vi "FPGA Main.vi"() -> ()   [LabVIEW 2024]
uses:
  <vilib>/eio/EIONode/EIONode.xnode
  <vilib>/rvi/eio/common/nirviEmuTemplateMethod_errors.vi
  Type Definitions/FPGA IO.ctl
  <vilib>/rvi/DataTransferAndStorage/Container/XNode/niFpgaContainer.xnode
  <vilib>/rvi/FIFO/Fifo_Resource/nirvififoEmulationRead.vi
  <vilib>/Platform/TimedLoop/XDataNode/wakeup.ctl
  <vilib>/Platform/TimedLoop/XDataNode/XDNodeRunTimeDep.lvlib
  <vilib>/Platform/TimedLoop/XDataNode/nitl_modes.ctl
  <vilib>/Platform/TimedLoop/XDataNode/timing_clust.ctl
  <vilib>/Platform/TimedLoop/XDataNode/XDataNode.xnode
  <vilib>/rvi/FIFO/Fifo_Resource/nirvififoEmulationWrite.vi
panel:
  in  "Enable Sinewave":bool
  in  "Sinewave Settings":T1={"Frequency (periods/tick)"=0.0, "Phase offset (periods)"=0.0, "Scale factor"=0.999969482421875, "Amplitude offset"=0.0}
  in  "Desired loop rate (ticks)":u32=2666666 caption="Update Interval (Ticks)"
  out "Actual loop rate":u32
  out "Sampling rate achieved?":bool
  out "Measured Period (Ticks)":u32
  out "Low Period (Ticks)":u32
  out "High Period (Ticks)":u32
  in  "Enable PWM":bool
  in  "Squarewave Settings":T2={"Frequency (periods/tick)"=0.0, "Phase offset (periods)"=0.0, "duty cycle (periods)"=0.5}
  in  "Initialize":bool
  in  "Voltage Out":fxp<+/-,20,5> format="%#.3g"
  in  "DO2":bool
  in  "DO1":bool
  in  "STOP FPGA":bool
  out "Potentiometer":fxp<+,18,3> format="%#.14g"
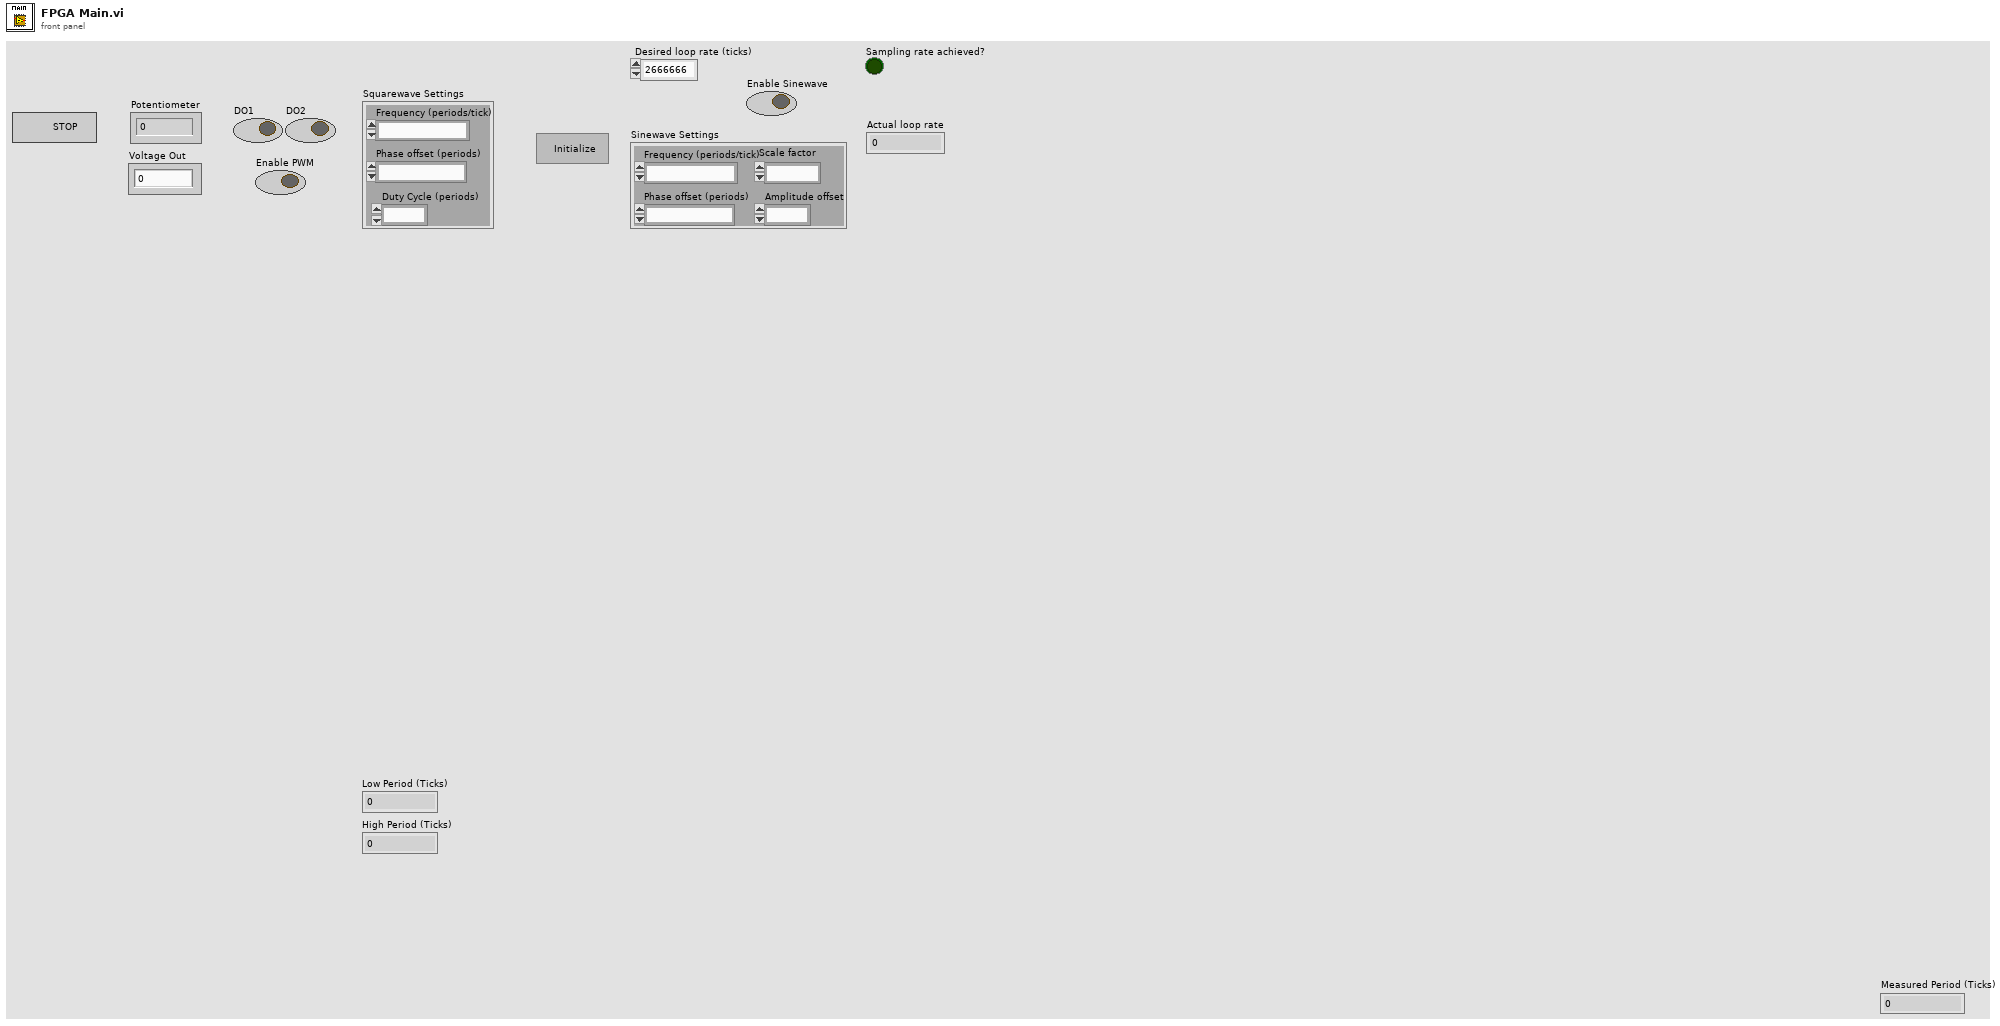
[diagram p1: front panel]
types:
  T1 = cluster{"Frequency (periods/tick)":fxp<+,32,0>, "Phase offset (periods)":fxp<+,32,0>, "Scale factor":fxp<+/-,16,1>, "Amplitude offset":fxp<+/-,16,16>}
  T2 = cluster{"Frequency (periods/tick)":fxp<+,32,0>, "Phase offset (periods)":fxp<+,32,0>, "duty cycle (periods)":fxp<+,32,0>}
  T3 = typedef "FPGA IO.ctl" = cluster{"DO1":bool, "DO2":bool, "Voltage Out":fxp<+/-,20,5>, "Crank Angle":fxp<+,18,3>, "Enable PWM":bool, "Enable Sinewave":bool}
  T4 = cluster{"DO1":bool, "DO2":bool, "Voltage Out":bool, "Crank Angle":bool, "Enable PWM":bool, "Enable Sinewave":bool}
  T5 = typedef "XDNodeRunTimeDep.lvlib/timing_clust.ctl" = cluster{"Expected End [f-1]":u64, "Actual End [f-1]":u64, "Finished Late? [f-1]":bool, "Expected End [i-1]":u64, "Actual End [i-1]":u64, "Finished Late? [i-1]":bool, "Expected Start [i]":u64, "Actual Start [i]":u64, "Expected Start [f]":u64, "Actual Start [f]":u64, "Source Name":string, "Structure Name":string, "Period":i64, "Deadline":i64, "Offset":i64, "Start":i64, "Priority":i32, "Timeout":i32, "Mode":T6, "Wakeup Reason":T7, "Error":errorcluster, "Source Type":string, "Secondary Source Type":string, "Global End Time":u64, "Global Start Time":u64, "Frame Duration":u64, "Iteration Duration":u64, "Assigned CPU":i32, "I/O Scan Engine Mode":u32}
  T6 = typedef "XDNodeRunTimeDep.lvlib/nitl_modes.ctl" = enum32{"No Change", "Process missed periods, maintain original phase", "Discard missed periods, maintain original phase", "Process missed periods, ignore original phase", "Discard missed periods, ignore original phase"}
  T7 = typedef "XDNodeRunTimeDep.lvlib/wakeup.ctl" = enum32{"Normal", "Aborted", "Asynchronous wakeup", "Timing source error", "Timed loop error", "Timeout"}
  T8 = cluster{"DO1":bool, "DO2":bool, "Voltage Out":fxp<+/-,20,5>, "Crank Angle":fxp<+,18,3>, "Enable PWM":bool, "Enable Sinewave":bool}
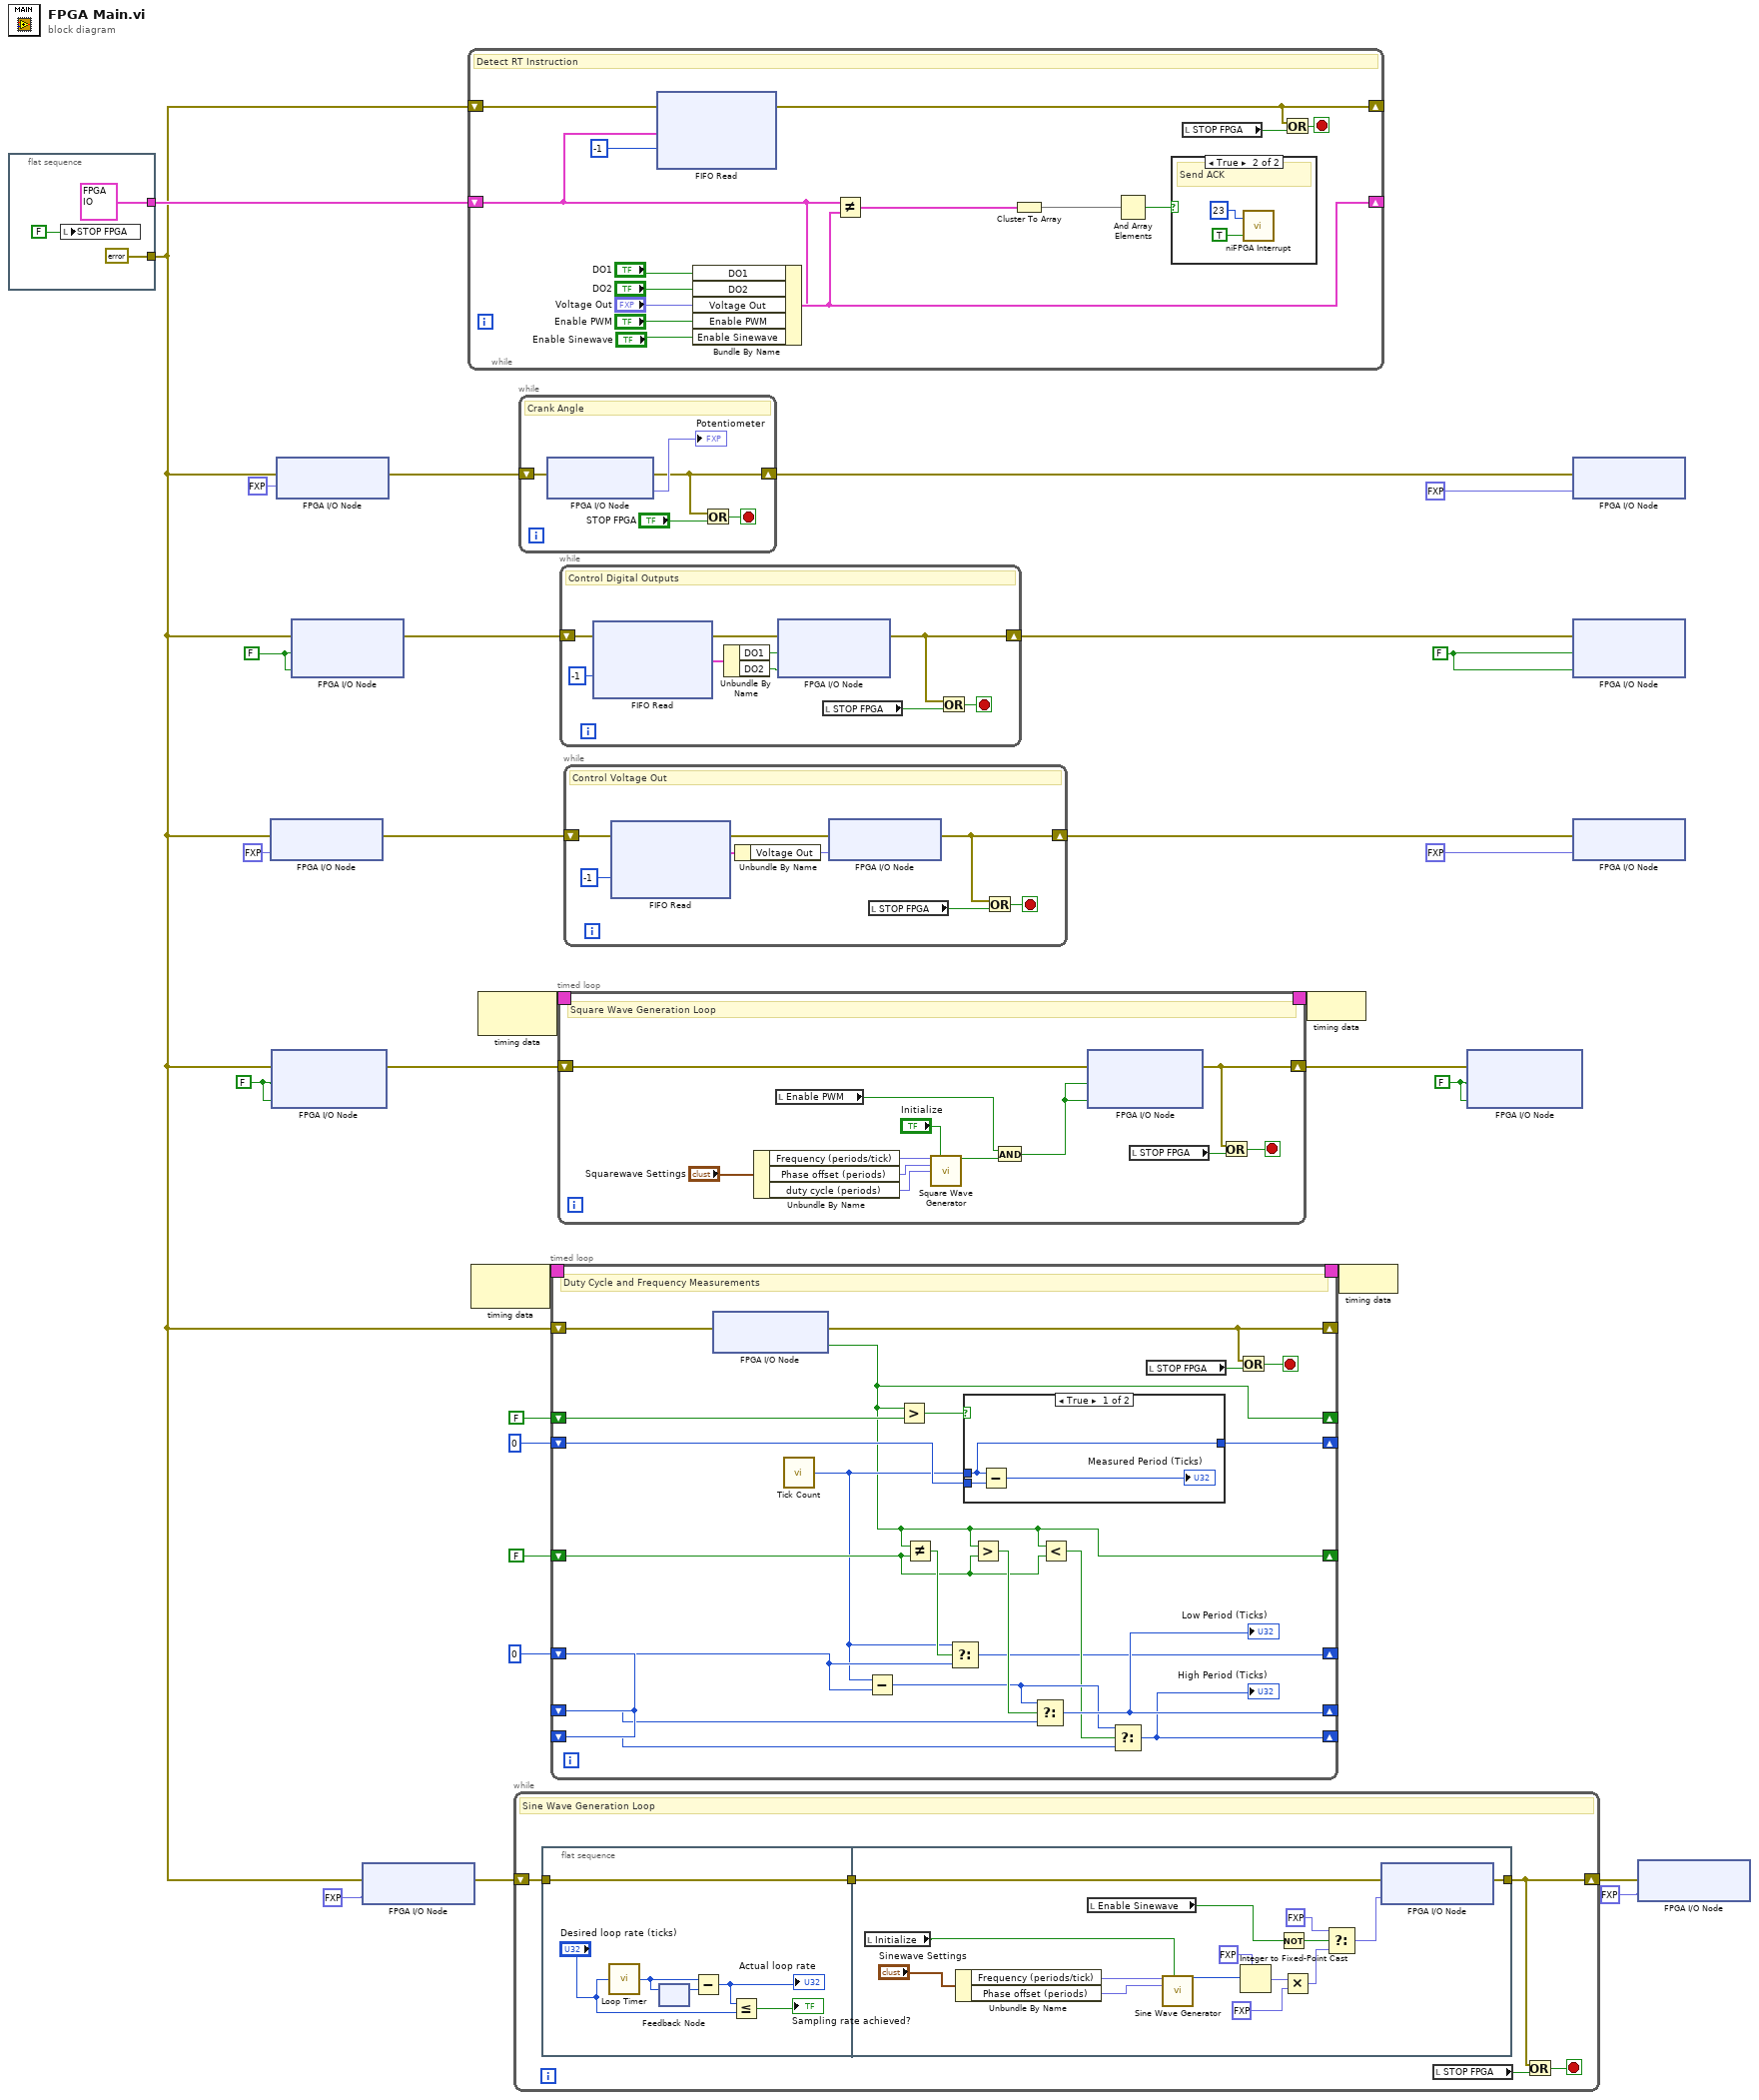
[diagram p0: block diagram]
diagram:
  w11 = u32 0 ("Tick Count(Ticks)")
  w2 = FALSE ("Mod3/DO0")
  w1 = FALSE ("Mod3/DO3")
  w22 = FALSE ("NI-9472/DO3")
  w19 = FALSE ("NI-9472/DO3")
  n1 = flat-sequence {
    tunnel: [errorcluster {"status"=FALSE, "code"=0, "source"=""} ("error in")] -> w6
    tunnel: [T3 {"DO1"=FALSE, "DO2"=FALSE, "Voltage Out"=0.0, "Crank Angle"=0.0, "Enable PWM"=FALSE, "Enable Sinewave"=FALSE} ("Cluster")] -> w20
    frame #0 {
      n2 = local write "STOP FPGA"(FALSE ("STOP FPGA")) -> ()
    }
  }
  n3 = xnode "FPGA I/O Node"("error in"=w6, "NI-9263/AO0"=fxp<+/-,20,5> 0.0) -> ("error out"=w25:errorcluster)  [unwired: 1 in, 1 out]
  n4 = xnode "FPGA I/O Node"("error in"=w6, "NI-9474/DO0"=w1, "NI-9381/DIO0"=w1) -> ("error out"=w15:errorcluster)  [unwired: 2 in, 2 out]
  n5 = xnode "FPGA I/O Node"("error in"=w6, "NI-9381/AO0"=fxp<+,16,3> 5.0) -> ("error out"=w29:errorcluster)  [unwired: 1 in, 1 out]
  n6 = xnode "FPGA I/O Node"("error in"=w6, "NI-9474/DO3"=w19, "NI-9474/DO7"=w19) -> ("error out"=w18:errorcluster)  [unwired: 2 in, 2 out]
  n7 = xnode "FPGA I/O Node"("error in"=w6, "NI-9263/AO1"=fxp<+/-,20,5> 0.0) -> ("error out"=w7:errorcluster)  [unwired: 1 in, 1 out]
  n8 = while {
    shift-right: [w46] -> _
    shift-left: w20 -> [w35]
    shift-right: [w40] -> _
    shift-left: w6 -> [w42]
    stop <- w39 stop-if-true
    # "Detect RT Instruction"
    n9 = xnode ("FIFO Read")("Element"=w35, "Timeout"=-1, "error in (no error)"=w42) -> ("error out"=w40:errorcluster)  [unwired: 1 in, 2 out]
    n10 = Bundle By Name(cluster=w35, "DO1"="DO1", "DO2"="DO2", "Voltage Out"="Voltage Out", "Enable PWM"="Enable PWM", "Enable Sinewave"="Enable Sinewave") -> (w46:T3)
    n11 = Not Equal?(x=w35, y=w46) -> (x != y?=w37:T4)
    n12 = Cluster To Array(cluster=w37) -> (array=w36:bool[])
    n13 = And Array Elements(Boolean array=w36) -> (logical AND=w45:bool)
    n14 = case shown="True" w45 {
      frame False {
      }
      frame True {
        # "Send ACK"
        n15 = call <vilib>:"niFPGA Interrupt.vi"("Wait Until Cleared (F)"=TRUE, "IRQ Number (0)"=u8 23) -> ()  [unwired: 1 in]
      }
    }
    n16 = local read "STOP FPGA"() -> (w41:bool)
    n17 = Or(x=w40, y=w41) -> (x .or. y?=w39:bool)
  }
  n18 = node-c288() -> (w13:T5)  [unwired: 1 in]
  n19 = node-c288() -> (w17:T5)  [unwired: 1 in]
  n20 = while {
    shift-right: [w51] -> w4
    shift-left: w7 -> [w55]
    stop <- w52 stop-if-true
    # "Sine Wave Generation Loop"
    n21 = flat-sequence {
      tunnel: w55 -> [w56]
      tunnel: [w56] -> w54
      tunnel: [w72] -> w51
      tunnel: w54 -> [w71]
      frame #0 {
        n22 = call "Loop Timer"("Count(Ticks)"="Desired loop rate (ticks)") -> ("Tick Count(Ticks)"=w61:u32)
        n23 = feedback-in #1(w61) -> ()
        n24 = feedback #1() -> (w60:u32)  [unwired: 1 out]
        n25 = Subtract(x=w61, y=w60) -> (x-y=w58:u32)
        "Actual loop rate" <- w58
        n26 = Less Or Equal?(x=w58, y="Desired loop rate (ticks)") -> (x <= y?=→"Sampling rate achieved?":bool)
      }
      frame #1 {
        n27 = local read "Initialize"() -> (w73:bool)
        n28 = Unbundle By Name("Sinewave Settings") -> ("Frequency (periods/tick)"=w76:fxp<+,32,0>, "Phase offset (periods)"=w75:fxp<+,32,0>)
        n29 = local read "Enable Sinewave"() -> (w69:bool)
        n30 = call "Sine Wave Generator"("frequency (periods/tick)"=w76, "reset"=w73, "phase offset (periods)"=w75) -> ("sine out"=w62:i16)  [unwired: 12 in]
        n31 = Integer to Fixed-Point Cast(fixed-point type=fxp<+/-,20,5> 0.0 ("NI-9263/AO1"), integer=w62) -> (fixed-point=w68:fxp<+/-,20,5>)
        n32 = Not(x=w69) -> (.not. x?=w70:bool)
        n33 = Multiply(x=w68, y=fxp<+/-,20,5> 10.0 ("NI-9263/AO1")) -> (x*y=w65:fxp<+/-,40,10>)
        n34 = Select(t=fxp<+/-,20,5> 0.0 ("NI-9263/AO1"), s=w70, f=w65) -> (s? t:f=w63:fxp<+/-,40,10>)
        n35 = xnode "FPGA I/O Node"("error in"=w71, "NI-9263/AO1"=w63) -> ("error out"=w72:errorcluster)  [unwired: 1 in, 1 out]
      }
    }
    n36 = local read "STOP FPGA"() -> (w53:bool)
    n37 = Or(x=w51, y=w53) -> (x .or. y?=w52:bool)
  }
  n38 = while {
    shift-right: [w77] -> w27
    shift-left: w29 -> [w81]
    stop <- w78 stop-if-true
    # "Crank Angle"
    n39 = xnode "FPGA I/O Node"("error in"=w81) -> ("error out"=w77:errorcluster, "NI-9381/AI0"=→"Potentiometer":fxp<+,18,3>)  [unwired: 1 in, 1 out]
    n40 = Or(x=w77, y="STOP FPGA") -> (x .or. y?=w78:bool)
  }
  n41 = timed-loop {
    shift-left: w11 -> [w93]
    shift-right: [w94] -> _
    shift-left: w11 -> [w99]
    shift-right: [w100] -> _
    shift-left: FALSE ("Input") -> [w96]
    shift-right: [w86] -> _
    shift-left: w11 -> [w101]
    shift-right: [w92] -> _
    timing: w13 -> [_]
    timing-out: [_] -> w12
    shift-right: [w86] -> _
    shift-left: FALSE ("Digital Signal A") -> [w91]
    shift-right: [w89] -> _
    shift-left: u32 0 ("Tick Count(Ticks)") -> [w90]
    shift-right: [w82] -> _
    shift-left: w6 -> [w85]
    stop <- w83 stop-if-true
    # "Duty Cycle and Frequency Measurements"
    n42 = xnode "FPGA I/O Node"("error in"=w85) -> ("error out"=w82:errorcluster, "NI-9381/DIO1"=w86:bool)  [unwired: 1 in, 1 out]
    n43 = call "Tick Count"() -> ("Tick Count(Ticks)"=w87:u32)
    n44 = Subtract(x=w87, y=w101) -> (x-y=w97:u32)
    n45 = Greater?(x=w86, y=w91) -> (0:w88:bool)
    n46 = Not Equal?(x=w86, y=w96) -> (x != y?=w102:bool)
    n47 = Select(t=w87, s=w102, f=w101) -> (s? t:f=w92:u32)
    n48 = case shown="True" w88 {
      tunnel: w87 -> [w103 _]
      tunnel: w90 -> [w104 w106]
      tunnel: [w103 w106] -> w89
      frame True {
        n49 = Subtract(x=w103, y=w104) -> (x-y=→"Measured Period (Ticks)":u32)
      }
      frame False {
      }
    }
    n50 = Greater?(x=w86, y=w96) -> (0:w98:bool)
    n51 = Select(t=w97, s=w98, f=w99) -> (s? t:f=w100:u32)
    "Low Period (Ticks)" <- w100
    n52 = Less?(x=w86, y=w96) -> (x < y?=w95:bool)
    n53 = Select(t=w97, s=w95, f=w93) -> (s? t:f=w94:u32)
    "High Period (Ticks)" <- w94
    n54 = local read "STOP FPGA"() -> (w84:bool)
    n55 = Or(x=w82, y=w84) -> (x .or. y?=w83:bool)
  }
  n56 = timed-loop {
    timing: w17 -> [_]
    timing-out: [_] -> w16
    shift-right: [w115] -> w14
    shift-left: w15 -> [w112]
    stop <- w114 stop-if-true
    # "Square Wave Generation Loop"
    n57 = Unbundle By Name("Squarewave Settings") -> ("Frequency (periods/tick)"=w119:fxp<+,32,0>, "Phase offset (periods)"=w118:fxp<+,32,0>, "duty cycle (periods)"=w117:fxp<+,32,0>)
    n58 = local read "Enable PWM"() -> (w110:bool)
    n59 = call "Square Wave Generator"("frequency (periods/tick)"=w119, "reset"="Initialize", "phase offset (periods)"=w118, "duty cycle (periods)"=w117) -> ("square wave out"=w113:bool)  [unwired: 11 in]
    n60 = And(x=w110, y=w113) -> (x .and. y?=w109:bool)
    n61 = xnode "FPGA I/O Node"("error in"=w112, "NI-9474/DO0"=w109, "NI-9381/DIO0"=w109) -> ("error out"=w115:errorcluster)  [unwired: 2 in, 2 out]
    n62 = local read "STOP FPGA"() -> (w116:bool)
    n63 = Or(x=w115, y=w116) -> (x .or. y?=w114:bool)
  }
  n64 = while {
    shift-right: [w125] -> w21
    shift-left: w18 -> [w129]
    stop <- w131 stop-if-true
    # "Control Digital Outputs"
    n65 = xnode ("FIFO Read")("Timeout"=-1, "error in (no error)"=w129) -> ("Element"=w128:T8, "error out"=w126:errorcluster)  [unwired: 1 in, 2 out]
    n66 = Unbundle By Name(w128) -> ("DO1"=w124:bool, "DO2"=w123:bool)
    n67 = xnode "FPGA I/O Node"("error in"=w126, "NI-9474/DO3"=w124, "NI-9474/DO7"=w123) -> ("error out"=w125:errorcluster)  [unwired: 2 in, 2 out]
    n68 = local read "STOP FPGA"() -> (w130:bool)
    n69 = Or(x=w125, y=w130) -> (x .or. y?=w131:bool)
  }
  n70 = while {
    shift-right: [w138] -> w23
    shift-left: w25 -> [w133]
    stop <- w139 stop-if-true
    # "Control Voltage Out"
    n71 = xnode ("FIFO Read")("Timeout"=-1, "error in (no error)"=w133) -> ("Element"=w136:T8, "error out"=w132:errorcluster)  [unwired: 1 in, 2 out]
    n72 = Unbundle By Name(w136) -> ("Voltage Out"=w134:fxp<+/-,20,5>)
    n73 = xnode "FPGA I/O Node"("error in"=w132, "NI-9263/AO0"=w134) -> ("error out"=w138:errorcluster)  [unwired: 1 in, 1 out]
    n74 = local read "STOP FPGA"() -> (w137:bool)
    n75 = Or(x=w138, y=w137) -> (x .or. y?=w139:bool)
  }
  n76 = node-c288(w16) -> ()
  n77 = node-c288(w12) -> ()
  n78 = xnode "FPGA I/O Node"("error in"=w14, "NI-9474/DO0"=w2, "NI-9381/DIO0"=w2) -> ()  [unwired: 2 in, 3 out]
  n79 = xnode "FPGA I/O Node"("error in"=w27, "NI-9381/AO0"=fxp<+,16,3> 0.0) -> ()  [unwired: 1 in, 2 out]
  n80 = xnode "FPGA I/O Node"("error in"=w21, "NI-9474/DO3"=w22, "NI-9474/DO7"=w22) -> ()  [unwired: 2 in, 3 out]
  n81 = xnode "FPGA I/O Node"("error in"=w23, "NI-9263/AO0"=fxp<+/-,20,5> 0.0) -> ()  [unwired: 1 in, 2 out]
  n82 = xnode "FPGA I/O Node"("error in"=w4, "NI-9263/AO1"=fxp<+/-,20,5> 0.0) -> ()  [unwired: 1 in, 2 out]
